vi "read result.vi"(10 "sent command":string, 11 "reference":refnum<visa-resource-name>) -> (0 "result string":string, 3 "dup VISA resource name":refnum<visa-resource-name>)   [LabVIEW 2010]
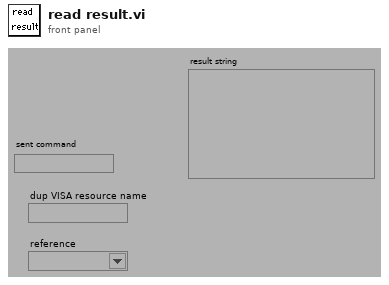
[diagram p1: front panel]
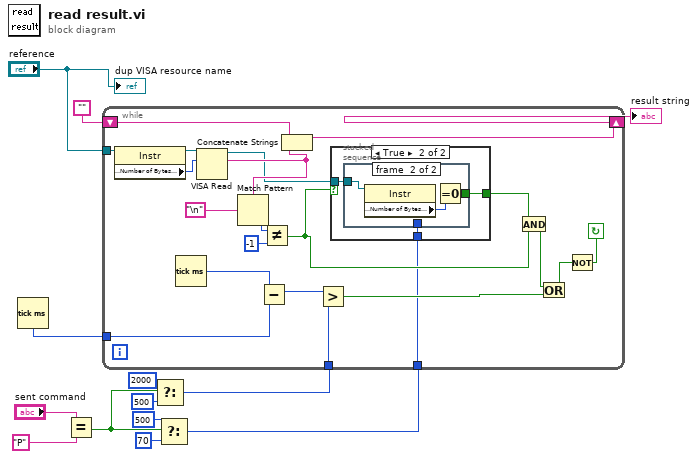
[diagram p0: block diagram]
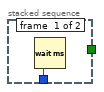
[diagram p3: hidden frame]
diagram:
  n1 = Tick Count (ms)() -> (millisecond timer value=w11:u32)
  n2 = Equal?(x="sent command", y="P") -> (x = y?=w3:bool)
  n3 = Select(t=2000, s=w3, f=500) -> (s? t:f=w2:i32)
  n4 = Select(t=500, s=w3, f=70) -> (s? t:f=w8:i32)
  n5 = while {
    tunnel: w2 -> [w19]
    tunnel: w8 -> [w20]
    tunnel: w11 -> [w22]
    shift-left: "" -> [w33]
    shift-right: [w34] -> w12
    tunnel: "reference" -> [w18]
    stop <- w27 continue-if-true
    n6 = property class="Instr"(reference=w18) -> (reference out=w17:refnum<visa-resource-name>, "Serial Settings:Number of Bytes at Serial Port"=w15:u32)  [unwired: 1 in, 1 out]
    n7 = Tick Count (ms)() -> (millisecond timer value=w21:u32)
    n8 = VISA Read(VISA resource name=w17, byte count=w15) -> (VISA resource name out=w14:refnum<visa-resource-name>, read buffer=w16:string)  [unwired: 1 in, 2 out]
    n9 = Match Pattern(string=w16, regular expression="\n") -> (offset past match=w30:i32)  [unwired: 1 in, 3 out]
    n10 = Subtract(x=w21, y=w22) -> (x-y=w32:u32)
    n11 = Not Equal?(x=w30, y=-1) -> (x != y?=w25:bool)
    n12 = Concatenate Strings(w33, w16) -> (w34:string)
    n13 = Greater?(x=w32, y=w19) -> (0:w26:bool)
    n14 = case shown="True" w25 {
      selector: w25 -> [w35 _]
      tunnel: w14 -> [_ w38]
      tunnel: [w35 w37] -> w28
      tunnel: w20 -> [_ w36]
      frame False {
      }
      frame True {
        n15 = stacked-sequence {
          tunnel: w38 -> [_ w41]
          tunnel: [_ w42] -> w37
          tunnel: w36 -> [w39 _]
          frame #0 {
            n16 = Wait (ms)(milliseconds to wait=w39) -> ()  [unwired: 1 out]
          }
          frame #1 {
            n17 = property class="Instr"(reference=w41) -> ("Serial Settings:Number of Bytes at Serial Port"=w40:u32)  [unwired: 1 in, 2 out]
            n18 = Equal To 0?(x=w40) -> (x = 0?=w42:bool)
          }
        }
      }
    }
    n19 = And(x=w28, y=w25) -> (x .and. y?=w24:bool)
    n20 = Or(x=w24, y=w26) -> (x .or. y?=w23:bool)
    n21 = Not(x=w23) -> (.not. x?=w27:bool)
  }
  "result string" <- w12
  "dup VISA resource name" <- "reference"
